vi "RSZVB Set Virtual Transform Port Pair Circuit Model.vi"(6 "Circuit Model (Serial Cs, shunt L)":i32(ring)=5 items=["File import, no circuit model", "Serial Touchstone (.s2p) data, shunt L", "Serial Touchstone (.s2p) data, shunt C", "Shunt L, serial Touchstone (.s2p) data", "Shunt C, serial Touchstone (.s2p) data", "Serial Cs, shunt L", "Serial Ls, shunt C", "Serial Cs, shunt C", "Serial Ls, shunt L", "Shunt L, serial Cs", "Shunt C, serial Ls", "Shunt C, serial Cs", "Shunt L, serial Ls"], 7 "Port Pair (1)":i32=1, 8 "error in (no error)":errorcluster {"code" format="%.0x"}, 9 "Function Type (Deembedding)":i32(ring) items=["Deembedding", "Embedding"], 10 "Channel (1)":i32=1, 11 "VISA session":refnum<visa-resource-name>) -> (0 "error out":errorcluster {"code" format="%.0x"}, 3 "dup VISA session":refnum<visa-resource-name>)   [LabVIEW 2011]
doc: "This VI selects the circuit model for port pair deembedding/embedding.\n\nRemote-control command(s):\nCALCulate<Ch>:TRANsform:VNETworks:PPAir:DEEMbedding<List_idx>:TNDefinition\nFIMPort | STSL | STSC | SLST | SCST | CSSL | LSSC | CSSC | LSSL | SLCS | SCLS | SCCS | SLLS \nCALCulate<Ch>:TRANsform:VNETworks:PPAir:EMBedding<List_idx>:TNDefinition\nFIMPort | STSL | STSC | SLST | SCST | CSSL | LSSC | CSSC | LSSL | SLCS | SCLS | SCCS | SLLS"
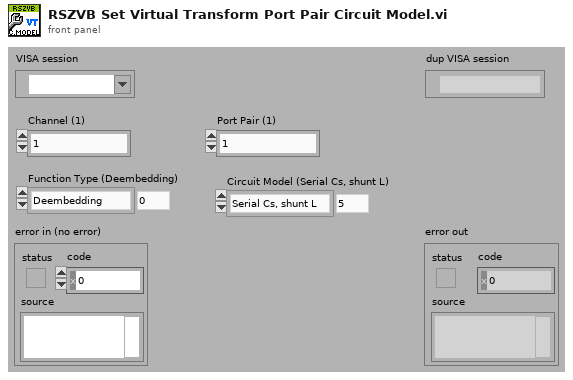
[diagram p1: front panel]
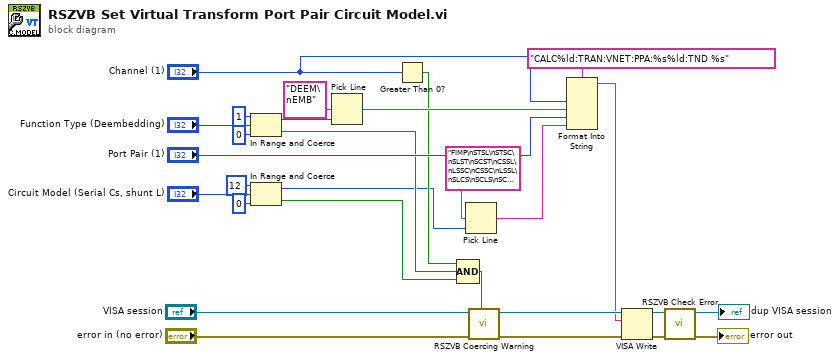
[diagram p0: block diagram]
diagram:
  n1 = In Range and Coerce(upper limit=1, x="Function Type (Deembedding)", lower limit=0) -> (coerced(x)=w19:i32, In Range?=w12:bool)
  n2 = In Range and Coerce(upper limit=12, x="Circuit Model (Serial Cs, shunt L)", lower limit=0) -> (coerced(x)=w7:i32, In Range?=w11:bool)
  n3 = Pick Line(multi-line string="DEEM\nEMB", line index=w19) -> (output string=w18:string)  [unwired: 1 in]
  n4 = Greater Than 0?(x="Channel (1)") -> (x > 0?=w13:bool)
  n5 = Compound Arithmetic op=AND(w13, w12, w11) -> (w2:bool)
  n6 = Pick Line(multi-line string="FIMP\nSTSL\nSTSC\nSLST\nSCST\nCSSL\nLSSC\nCSSC\nLSSL\nSLCS\nSCLS\nSCCS\nSLLS", line index=w7) -> (output string=w8:string)  [unwired: 1 in]
  n7 = call "RSZVB Coercing Warning.vi"("In Range?"=w2, "error in (no error)"="error in (no error)", "VISA session"="VISA session") -> ("error out"=w24:errorcluster, "dup VISA session"=w25:refnum<visa-resource-name>)  [unwired: 7 in]
  n8 = Format Into String(format string="CALC%ld:TRAN:VNET:PPA:%s%ld:TND %s", "Channel (1)", w18, "Port Pair (1)", w8) -> (resulting string=w17:string)  [unwired: 2 in, 1 out]
  n9 = VISA Write(VISA resource name=w25, write buffer=w17, error in (no error)=w24) -> (VISA resource name out=w28:refnum<visa-resource-name>, error out=w27:errorcluster)  [unwired: 1 out]
  n10 = call "RSZVB Check Error.vi"("error in (no error)"=w27, "VISA session"=w28) -> ("error out"=→"error out":errorcluster, "dup VISA session"=→"dup VISA session":refnum<visa-resource-name>)  [unwired: 8 in]
